vi "Import DMA Channels RTM.vi"(8 "error in (no error)":errorcluster, 11 "Node Ptr":u64 format="%.0x") -> (0 "error out":errorcluster)   [LabVIEW 2019, in "FPGA Addon System Explorer.lvlib"]
uses:
  FPGA Addon System Explorer.lvlib
  Shared/FG Action.ctl
  Shared/Constants.vi
  <vilib>/NI VeriStand/Custom Device API/NI VeriStand - Get Item Property.vi
  <vilib>/NI VeriStand/Custom Device API/Get Item Property (U32).vi
  <vilib>/NI VeriStand/Custom Device API/Get Item Property (Double).vi
  <vilib>/NI VeriStand/Custom Device API/NI VeriStand - Set Item Property.vi
  <vilib>/NI VeriStand/Custom Device API/Set Item Property (U32).vi
  <vilib>/NI VeriStand/Custom Device API/Set Item Property (Double).vi
  Shared/FPGA Addon Shared.lvlib
  <vilib>/NI VeriStand/Custom Device Tools/Custom Device Utility Library/Custom Device Utility Library.lvlib
  <vilib>/NI VeriStand/Custom Device API/Custom Device API.lvlib
panel:
  in  "Tag":string
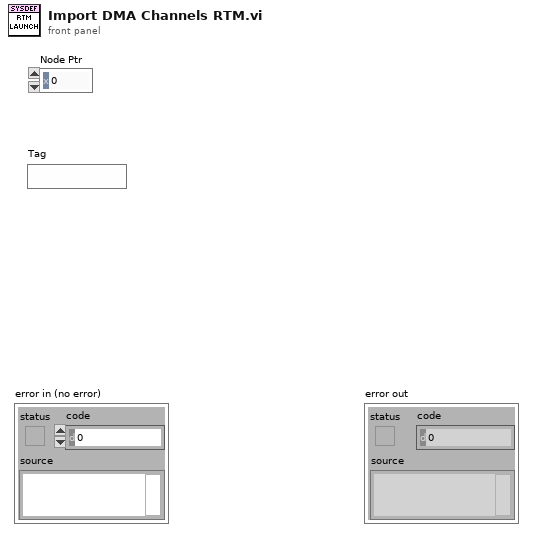
[diagram p1: front panel]
types:
  T1 = typedef "FPGA Addon Shared.lvlib/FG Action.ctl" = enum8{"GET", "SET"}
  T2 = typedef "Custom Device API.lvlib/Custom Device Item Ref.ctl" = u64
  T3 = typedef "FPGA Addon Shared.lvlib/DMA Settings.ctl" = cluster{"Number of Channels":u8, "Delacing Scheme":T4, "Update Rate":u32, "dt":dbl, "Mode":T5, "Number of Samples":u32, "DMA Host Buffer":u32}
  T4 = typedef "FPGA Addon Shared.lvlib/Delacing Scheme.ctl" = enum8{"Interleaved", "Bitpacked"}
  T5 = typedef "FPGA Addon Shared.lvlib/DMA Acquisition Mode.ctl" = enum8{"Continuous", "Triggered Finite"}
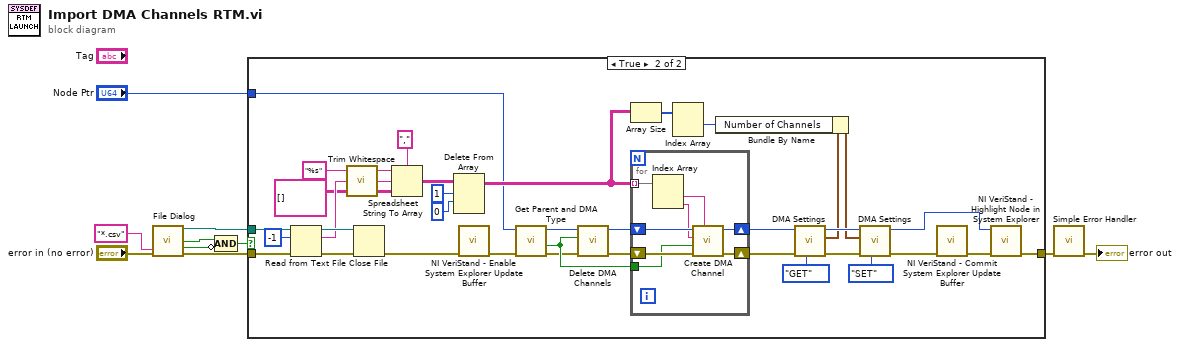
[diagram p0: block diagram]
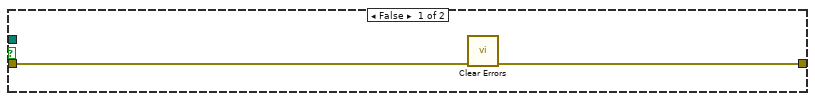
[diagram p2: hidden frame]
diagram:
  n1 = call "File Dialog"("error in"="error in (no error)", "pattern (all files)"="*.csv") -> ("selected path"=w9:path, "exists"=w7:bool, "cancelled"=w6:bool, "error out"=w8:errorcluster)  [unwired: 10 in]
  n2 = Compound Arithmetic op=AND(w7, invert w6) -> (w5:bool)
  n3 = case shown="True" w5 {
    tunnel: w9 -> [_ w48]
    tunnel: w8 -> [w12 w47]
    tunnel: "Node Ptr" -> [_ w20]
    tunnel: [w11 w17] -> w1
    frame False {
      n4 = call <vilib>:"Clear Errors.vi"("error in (no error)"=w12) -> ("error out"=w11:errorcluster)  [unwired: 5 in, 1 out]
    }
    frame True {
      n5 = Read from Text File(file (use dialog)=w48, count=-1, error in=w47) -> (refnum out=w44:refnum<file>, text=w43:string, error out=w46:errorcluster)  [unwired: 1 in, 1 out]
      n6 = call <vilib>:"Trim Whitespace.vi"("string"=w43) -> ("trimmed string"=w36:string)  [unwired: 1 in]
      n7 = Close File(refnum=w44, error in=w46) -> (error out=w14:errorcluster)  [unwired: 1 out]
      n8 = Spreadsheet String To Array(delimiter (Tab)=",", format string="%s", spreadsheet string=w36, array type (2D Dbl)=string[][] []) -> (array=w39:string[][])
      n9 = Delete From Array(array=w39, length=1, index (row)=0 ("index")) -> (array with subset deleted=w22:string[][])  [unwired: 1 in, 1 out]
      n10 = call <vilib>:"NI VeriStand - Enable System Explorer Update Buffer.vi"("error in (no error)"=w14) -> ("error out"=w13:errorcluster)  [unwired: 10 in]
      n11 = call "Get Parent and DMA Type.vi"("error in (no error)"=w13, "Node Ptr"=w20) -> ("error out"=w29:errorcluster, "Input?"=w35:bool, "Item Ref out"=w30:T2)  [unwired: 6 in, 1 out]
      n12 = call "Delete DMA Channels.vi"("error in (no error)"=w29, "Input?"=w35, "Item Ref in"=w30) -> ("error out"=w31:errorcluster, "Section Ref out"=w32:T2)  [unwired: 7 in]
      n13 = Array Size(array=w22) -> (size(s)=w21:i32[])
      n14 = for {
        shift-right: [w54] -> w33
        shift-left: w31 -> [w56]
        shift-right: [w53] -> w34
        shift-left: w32 -> [w55]
        tunnel: w35 -> [w52]
        tunnel: w22 -> [w51] mode=indexing
        n15 = Index Array(array=w51) -> (element #1=w50:string, element #2=w49:string)  [unwired: 2 in]
        n16 = call "Create DMA Channel.vi"("Original Name"=w50, "error in (no error)"=w56, "Input?"=w52, "Name"=w49, "Section Ref in"=w55) -> ("error out"=w54:errorcluster, "Parent Ref out"=w53:T2)  [unwired: 5 in]
      }
      n17 = Index Array(array=w21) -> (element #1=w19:i32)  [unwired: 2 in, 1 out]
      n18 = call "DMA Settings.vi"("Action"=FG_Action."GET", "error in (no error)"=w33, "Item Ref"=w34) -> ("error out"=w26:errorcluster, "DMA Settings"=w24:T3, "Item Ref out"=w25:T2)  [unwired: 6 in]
      n19 = Bundle By Name(cluster=w24, "Number of Channels"=w19) -> (w23:T3)
      n20 = call "DMA Settings.vi"("Action"=FG_Action."SET", "error in (no error)"=w26, "DMA Settings"=w23, "Item Ref"=w25) -> ("error out"=w16:errorcluster, "Item Ref out"=w18:T2)  [unwired: 5 in, 1 out]
      n21 = call <vilib>:"NI VeriStand - Commit System Explorer Update Buffer.vi"("error in (no error)"=w16) -> ("error out"=w15:errorcluster)  [unwired: 10 in]
      n22 = call <vilib>:"NI VeriStand - Highlight Node in System Explorer.vi"("error in (no error)"=w15, "Item Ref in"=w18) -> ("error out"=w17:errorcluster)  [unwired: 8 in, 1 out]
    }
  }
  n23 = call <vilib>:"Simple Error Handler.vi"("error in (no error)"=w1) -> ("error out"=→"error out":errorcluster)  [unwired: 4 in, 4 out]
